vi "LastElem.vi"(11 "X":dbl[](array[numeric])) -> (3 "Numeric Control":dbl)   [LabVIEW 2014, in "Manipulator.lvclass"]
uses:
  Manipulator.lvclass
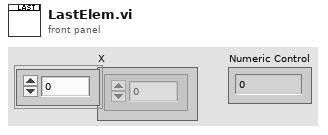
[diagram p1: front panel]
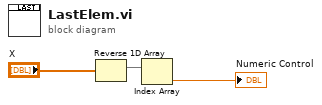
[diagram p0: block diagram]
diagram:
  n1 = Reverse 1D Array(array="X") -> (reversed array=w2:dbl[])
  n2 = Index Array(array=w2) -> (element=→"Numeric Control":dbl)  [unwired: 1 in]
